vi "example_00_load_class.vi"() -> ()   [LabVIEW 2015, in "lv-dialog.lvlib" / "v1.lvlib"]
uses:
  v1.lvlib
  lv-dialog-interfaces/public/api/v1/v1.lvclass
  public/_subvis/advanced/load_class-file.vi
  public/_subvis/advanced/load_class-class.vi
panel:
  in  "selection":enum32{"File/Filepath", "Builtin Class"}(radio)
  out "error":errorcluster
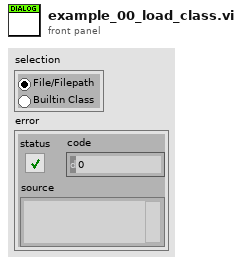
[diagram p1: front panel]
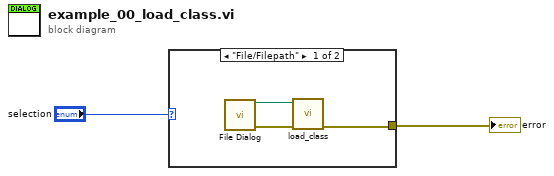
[diagram p0: block diagram]
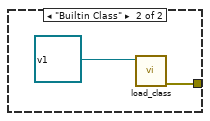
[diagram p2: hidden frame]
diagram:
  n1 = case shown="\"File/Filepath\"" "selection" {
    tunnel: [w3 w6] -> w2
    frame "File/Filepath" {
      n2 = call "File Dialog"() -> ("selected path"=w5:path, "error out"=w4:errorcluster)  [unwired: 12 in, 2 out]
      n3 = call-poly "load_class.vi"("error in (no error)"=w4, "class_path"=w5) -> ("error out"=w3:errorcluster)  [unwired: 9 in]
    }
    frame "Builtin Class" {
      n4 = call-poly "load_class.vi"("class"=refnum<class "v1.lvclass"> refnum ("lv-dialog-interfaces.lvlib:v1.lvclass")) -> ("error out"=w6:errorcluster)  [unwired: 10 in]
    }
  }
  "error" <- w2
